vi "group Sync Write Add Param.vi"(7 "data_length":u16, 9 "data":u32, 10 "id":u8, 11 "group_num":i32) -> (3 "function return":u8)   [LabVIEW 2015, in "dxl_x86_c.lvlib"]
doc: "WINDECLSPEC uint8_t groupSyncWriteAddParam (int group_num, uint8_t id, uint32_t data, uint16_t data_length);"
uses:
  dxl_x86_c.lvlib
  dxl_x86_c.dll
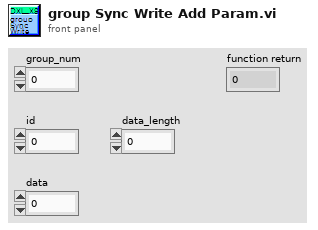
[diagram p1: front panel]
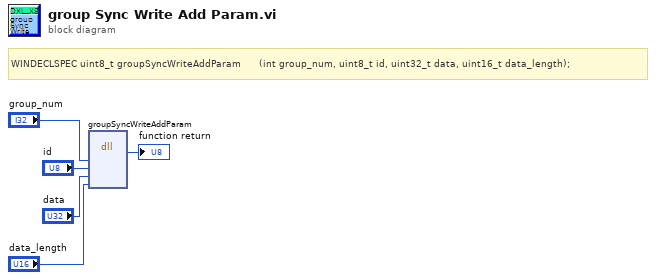
[diagram p0: block diagram]
diagram:
  # "WINDECLSPEC uint8_t groupSyncWriteAddParam      (int group_num, uint8_t id, uint32_t data, uint16_t data_length);"
  n1 = dll-call lib="C:/Users/Platform/Desktop/LabVIEW/dxl_x86_c.lvlib/dxl_x86_c.*" fn="groupSyncWriteAddParam"("group_num"="group_num", "id"="id", "data"="data", "data_length"="data_length") -> (→"function return":u8)  [unwired: 7 in, 2 out]
